vi "HotLotMSSQLNew.vi"() -> ()   [LabVIEW 2012]
uses:
  <vilib>/Utility/NIReport.llb/NI_report.lvclass
  <vilib>/addons/database/Connection.llb/DB Tools Open Connec (Path).vi
  Global1.vi
  <vilib>/addons/database/NI_Database_API.lvlib
  <vilib>/Utility/NIReport.llb/Excel/NI_Excel.lvclass
panel:
  out "error out 4":errorcluster
  out "Array":string[][](array[string])
  out "data":string
  in  "Cluster":T1
  out "error out":errorcluster
  out "String":string
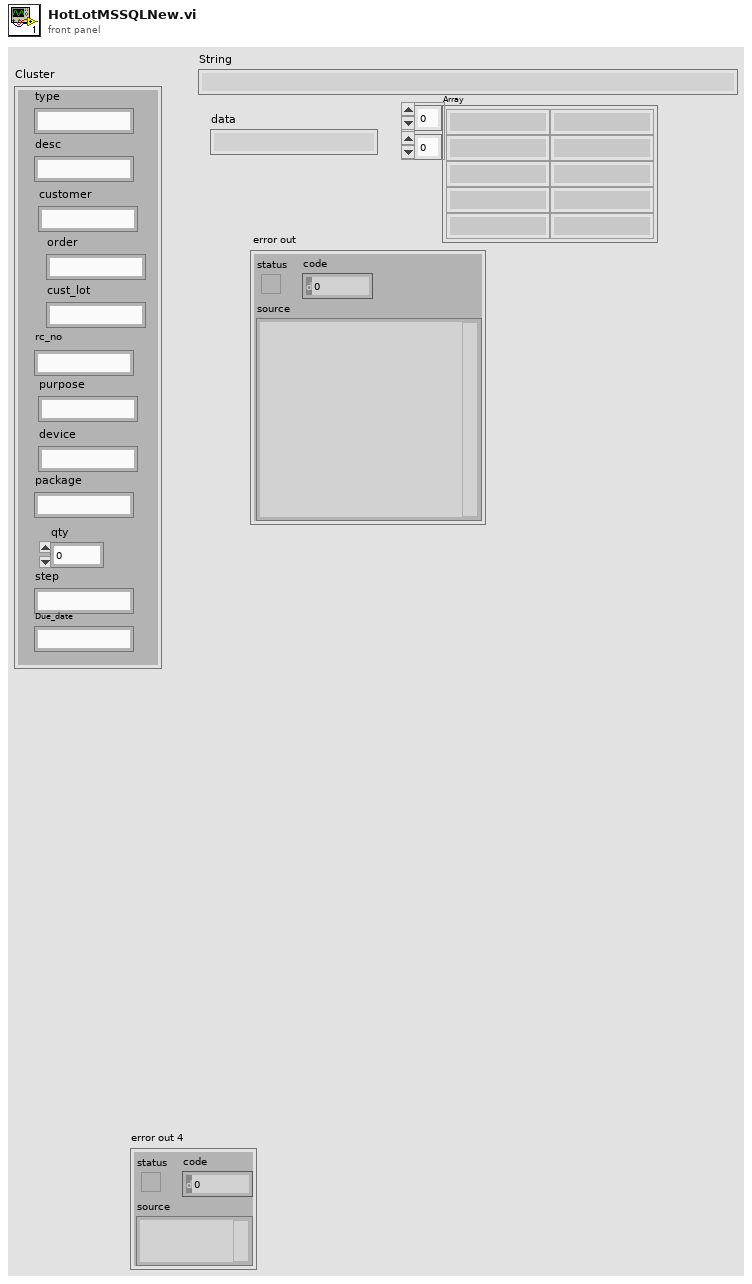
[diagram p1: front panel]
types:
  T1 = cluster{"type":string, "desc":string, "customer":string, "order":string, "cust_lot":string, "rc_no":string, "purpose":string, "device":string, "package":string, "qty":dbl, "step":string, "Due_date":string}
  T2 = enum16{"Standard Report", "HTML", "Word", "Excel"}
  T3 = typedef "NI_Database_API.lvlib/Conn ObjectReference.ctl" = refnum<k1>
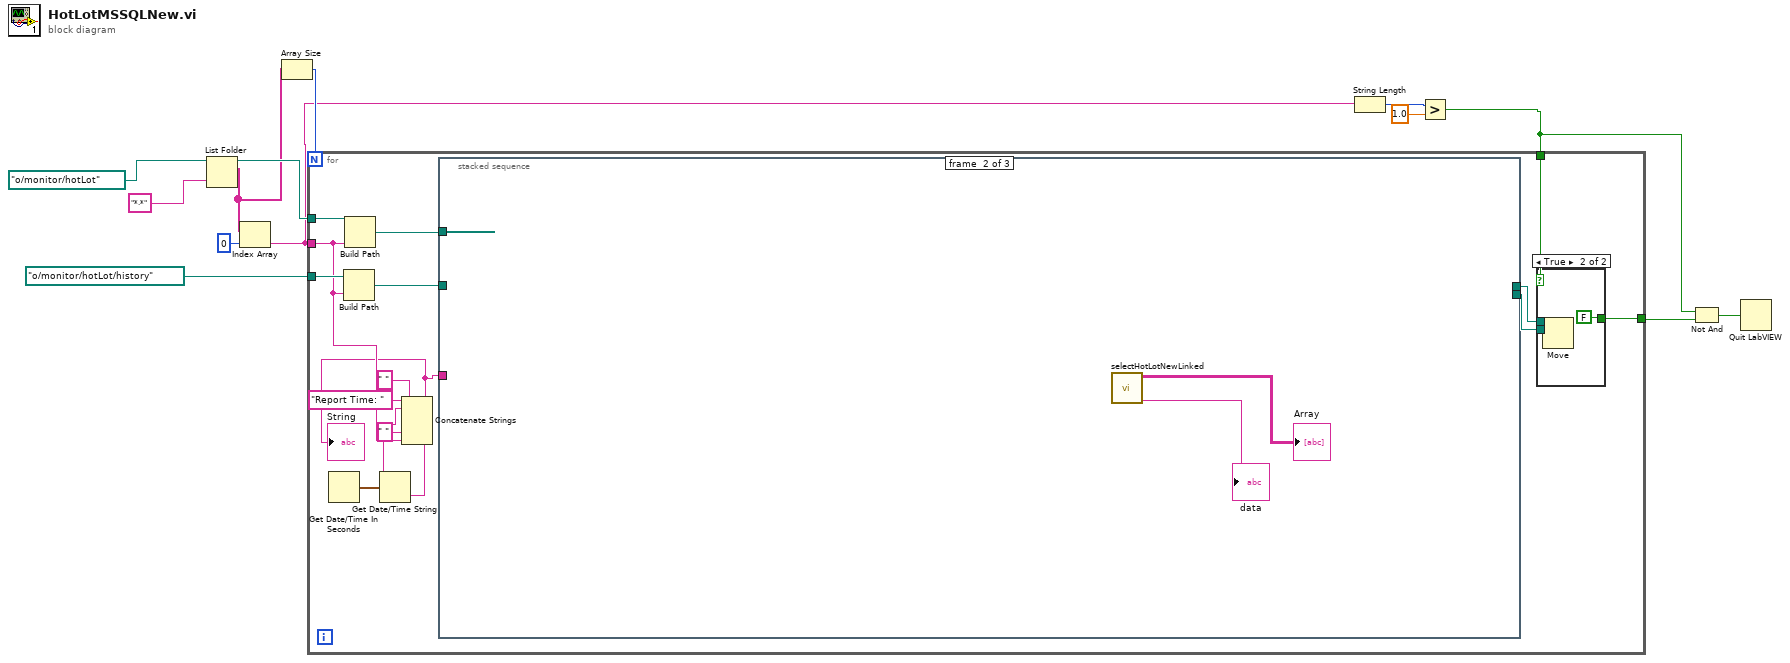
[diagram p0: block diagram]
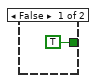
[diagram p2: hidden frame]
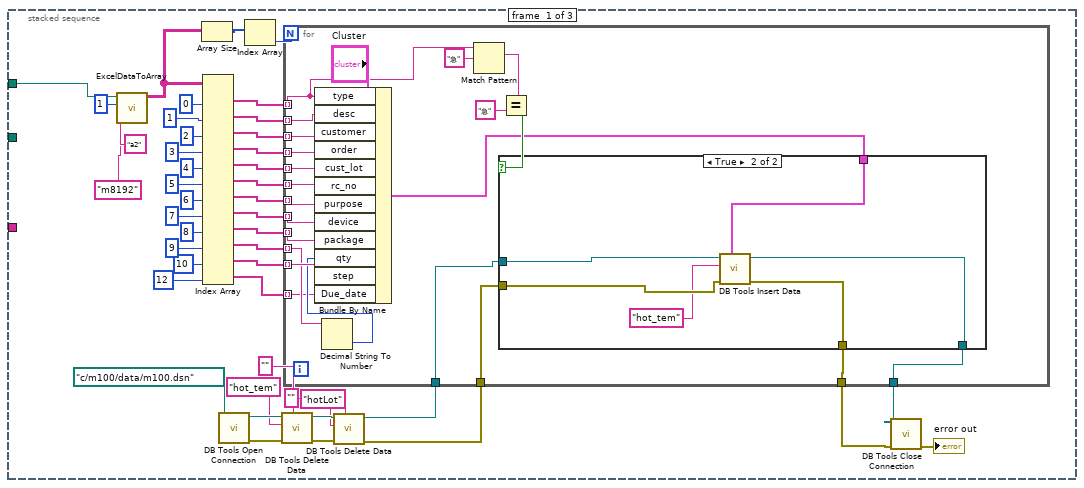
[diagram p3: hidden frame]
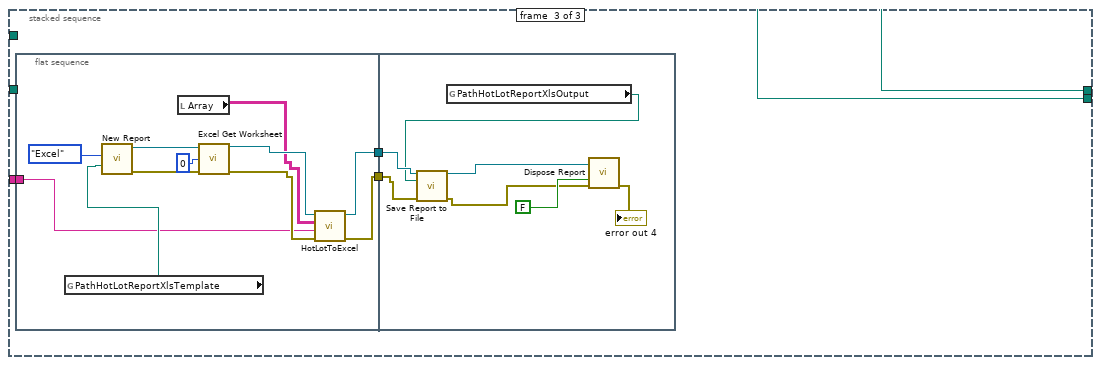
[diagram p5: hidden frame]
diagram:
  n1 = List Folder(path=path "o:/monitor/hotLot", pattern="*.*") -> (path out=w10:path, filenames=w9:string[])  [unwired: 2 in, 2 out]
  n2 = Index Array(array=w9, index=0) -> (element=w6:string)
  n3 = Array Size(array=w9) -> (size(s)=w12:i32)
  n4 = String Length(string=w6) -> (length=w4:i32)
  n5 = Greater?(x=w4, y=1.0) -> (0:w3:bool)
  n6 = for {
    N: w12 -> [_]
    tunnel: w6 -> [w16]
    tunnel: w10 -> [w29]
    tunnel: path "o:/monitor/hotLot/history" ("base path") -> [w27]
    tunnel: w3 -> [w23]
    tunnel: [w14] -> w2
    n7 = Get Date/Time In Seconds() -> (seconds since 1Jan1904=w22:timestamp)
    n8 = Build Path(base path=w27, name or relative path=w16) -> (appended path=w26:path)
    n9 = Build Path(base path=w29, name or relative path=w16) -> (appended path=w28:path)
    n10 = Get Date/Time String(seconds (now)=w22) -> (date string=w20:string, time string=w18:string)  [unwired: 2 in]
    n11 = Concatenate Strings("Report Time: " ("string"), w20, " " ("string"), w18, " " ("string"), w16) -> (w15:string)
    "String" <- w15
    n12 = stacked-sequence {
      tunnel: w28 -> [w46 _ w116]
      tunnel: w26 -> [_ _ w115]
      tunnel: [_ _ w116] -> w25
      tunnel: [_ _ w115] -> w24
      tunnel: w15 -> [_ _ w114]
      frame #0 {
        n13 = call "ExcelDataToArray.vi"("end cell"="m8192", "start cell"="a2", "sheet#"=1, "path"=w46) -> ("data"=w70:string[][])  [unwired: 6 in, 1 out]
        n14 = Array Size(array=w70) -> (size(s)=w74:i32[])
        n15 = Index Array(array=w70, index (col) #1=0 ("disabled index (col)"), index (col) #2=1 ("index (col)"), index (col) #3=2 ("index (col)"), index (col) #4=3 ("index (col)"), index (col) #5=4 ("index (col)"), index (col) #6=5 ("index (col)"), index (col) #7=6 ("index (col)"), index (col) #8=7 ("index (col)"), index (col) #9=8 ("index (col)"), index (col) #10=9 ("index (col)"), index (col) #11=10 ("index (col)"), index (col) #12=12 ("index (col)")) -> (element #1=w59:string[], element #2=w58:string[], element #3=w57:string[], element #4=w56:string[], element #5=w55:string[], element #6=w54:string[], element #7=w53:string[], element #8=w52:string[], element #9=w51:string[], element #10=w50:string[], element #11=w49:string[], element #12=w44:string[])  [unwired: 12 in]
        n16 = call-poly <vilib>:"DB Tools Open Connection.vi"("connection information"=path "c:/m100/data/m100.dsn") -> ("error out"=w42:errorcluster, "connection reference"=w43:T3)  [unwired: 7 in]
        n17 = Index Array(array=w74) -> (element=w73:i32)  [unwired: 1 in]
        n18 = call <vilib>:"DB Tools Delete Data.vi"("condition"="", "error in (no error)"=w42, "table"="hot_tem", "connection reference"=w43) -> ("error out"=w39:errorcluster, "connection reference out"=w40:T3)  [unwired: 6 in]
        n19 = call <vilib>:"DB Tools Delete Data.vi"("condition"="", "error in (no error)"=w39, "table"="hotLot", "connection reference"=w40) -> ("error out"=w37:errorcluster, "connection reference out"=w38:T3)  [unwired: 6 in]
        n20 = for {
          N: w73 -> [_]
          tunnel: w59 -> [w83] mode=indexing
          tunnel: w58 -> [w99] mode=indexing
          tunnel: w57 -> [w98] mode=indexing
          tunnel: w56 -> [w97] mode=indexing
          tunnel: w55 -> [w96] mode=indexing
          tunnel: w54 -> [w87] mode=indexing
          tunnel: w53 -> [w92] mode=indexing
          tunnel: w52 -> [w93] mode=indexing
          tunnel: w51 -> [w94] mode=indexing
          tunnel: w50 -> [w89] mode=indexing
          tunnel: w49 -> [w95] mode=indexing
          tunnel: [w85] -> w48
          tunnel: [w86] -> w47
          tunnel: w44 -> [w84] mode=indexing
          tunnel: w38 -> [w80]
          tunnel: w37 -> [w79]
          n21 = Decimal String To Number(string=w89) -> (number=w88:i32)  [unwired: 2 in, 1 out]
          n22 = Bundle By Name(cluster="Cluster", "type"=w83, "desc"=w99, "customer"=w98, "order"=w97, "cust_lot"=w96, "rc_no"=w87, "purpose"=w92, "device"=w93, "package"=w94, "qty"=w88, "step"=w95, "Due_date"=w84) -> (w90:T1)
          n23 = Match Pattern(string=w83, regular expression="急") -> (match substring=w81:string)  [unwired: 1 in, 3 out]
          n24 = Equal?(x=w81, y="急") -> (x = y?=w91:bool)
          n25 = case shown="True" w91 {
            tunnel: w90 -> [_ w104]
            tunnel: w80 -> [w102 w109]
            tunnel: w79 -> [w103 w108]
            tunnel: [w103 w105] -> w86
            tunnel: [w102 w106] -> w85
            frame False {
            }
            frame True {
              n26 = call <vilib>:"DB Tools Insert Data.vi"("data"=w104, "error in (no error)"=w108, "table"="hot_tem", "connection reference"=w109) -> ("error out"=w105:errorcluster, "connection reference out"=w106:T3)  [unwired: 6 in]
            }
          }
        }
        n27 = call <vilib>:"DB Tools Close Connection.vi"("error in (no error)"=w47, "connection reference"=w48) -> ("error out"=→"error out":errorcluster)  [unwired: 5 in]
      }
      frame #1 {
        n28 = call "selectHotLotNewLinked.vi"() -> ("data"=→"data":string, "Array"=→"Array":string[][])  [unwired: 10 in]
      }
      frame #2 {
        n29 = flat-sequence {
          tunnel: w114 -> [w117]
          tunnel: [w120] -> w113
          tunnel: [w119] -> w112
          tunnel: w113 -> [w130]
          tunnel: w112 -> [w129]
          frame #0 {
            n30 = global read "Global1.vi" "PathHotLotReportXlsTemplate"() -> (w123:path)
            n31 = call <vilib>:"New Report.vi"("report type"=T2."Excel" ("Report Type"), "template (empty)"=w123) -> ("report out"=w126:refnum<class "NI_report.lvclass">, "error out"=w125:errorcluster)  [unwired: 12 in]
            n32 = local read "Array"() -> (w118:string[][])
            n33 = call <vilib>:"Excel Get Worksheet.vi"("report in"=w126, "worksheet index (0)"=0, "error in (no error)"=w125) -> ("report out"=w122:refnum<class "NI_report.lvclass">, "error out"=w121:errorcluster)  [unwired: 11 in]
            n34 = call "HotLotToExcel.vi"("error in (no error)"=w121, "Header"=w117, "Input"=w118, "report in"=w122) -> ("error out"=w119:errorcluster, "report out"=w120:refnum<class "NI_report.lvclass">)  [unwired: 6 in]
          }
          frame #1 {
            n35 = global read "Global1.vi" "PathHotLotReportXlsOutput"() -> (w128:path)
            n36 = call-dynamic "Save Report to File.vi"("report in"=w130, "report file path"=w128, "error in (no error)"=w129) -> ("report out"=w131:refnum<class "NI_report.lvclass">, "error out"=w132:errorcluster)  [unwired: 11 in]
            n37 = call-dynamic "Dispose Report.vi"("report in"=w131, "save changes? (F)"=FALSE, "error in (no error)"=w132) -> ("error out"=→"error out 4":errorcluster)  [unwired: 12 in]
          }
        }
      }
    }
    n38 = case shown="True" w23 {
      tunnel: w25 -> [_ w33]
      tunnel: w24 -> [_ w32]
      tunnel: [TRUE FALSE] -> w14
      frame False {
      }
      frame True {
        n39 = Move(source path=w33, 10:w32) -> ()  [unwired: 3 in, 3 out]
      }
    }
  }
  n40 = Not And(1:w2, 2:w3) -> (0:w1:bool)
  n41 = Quit LabVIEW(quit? (T)=w1) -> ()
